vi "CloseTIFF.vi"(8 "error in (no error)":errorcluster, 11 "TIFF File Ref":i32) -> (0 "error out":errorcluster)   [LabVIEW 2012]
uses:
  VisualCPP/LabTIFF/Release/LabTIFF.dll
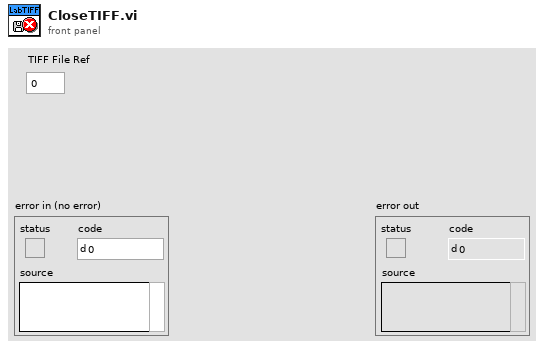
[diagram p1: front panel]
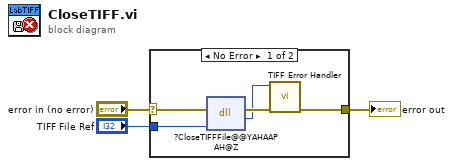
[diagram p0: block diagram]
diagram:
  n1 = case shown="No Error" "error in (no error)" {
    selector: "error in (no error)" -> [w8 w9]
    tunnel: "TIFF File Ref" -> [w7 _]
    tunnel: [w4 w9] -> w1
    frame No Error {
      n2 = dll-call lib="C:/Users/Ludo/Programming/Tests/TIFFManagement_test/LabTIFF/VisualCPP/LabTIFF/Release/LabTIFF.dll" fn="?CloseTIFFFile@@YAHAAPAH@Z"(error in=w8, "File Reference"=w7) -> (error out=w6:errorcluster, "error"=w5:i32)  [unwired: 3 in, 1 out]
      n3 = call "TIFF Error Handler.vi"("error in (no error)"=w6, "TIFF DLL error"=w5) -> ("error out"=w4:errorcluster)  [unwired: 9 in]
    }
    frame Error {
    }
  }
  "error out" <- w1
